vi "Merge Driver Call by Reference Error.vi"(8 "driver name":string, 10 "called vi error":errorcluster, 11 "call by ref error":errorcluster) -> (2 "error out":errorcluster)   [LabVIEW 2020, in "MeasurementLink Instrument.lvlib" / "ISession Factory.lvclass"]
uses:
  ISession Factory.lvclass
  MeasurementLink Measurement Server/Helpers/Error Strings Global Internal.vi
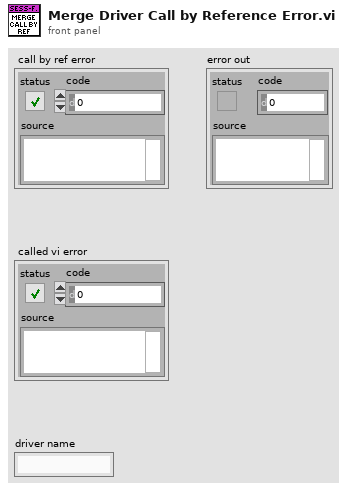
[diagram p1: front panel]
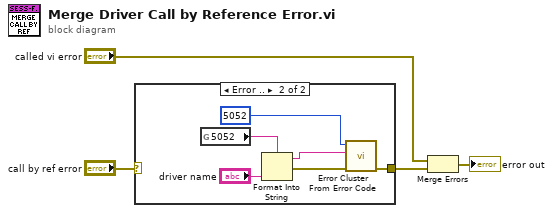
[diagram p0: block diagram]
diagram:
  n1 = case shown="Error .." "call by ref error" {
    selector: "call by ref error" -> [w5 _]
    tunnel: [w5 w6] -> w2
    frame No Error {
    }
    frame Error {
      n2 = global read "Error Strings Global Internal.vi" "5052"() -> (w9:string)
      n3 = Format Into String(format string=w9, "driver name") -> (resulting string=w10:string, error out=w11:errorcluster)  [unwired: 2 in]
      n4 = call <vilib>:"Error Cluster From Error Code.vi"("error in (no error)"=w11, "error message (\"\")"=w10, "error code (0)"=5052) -> ("error out"=w6:errorcluster)  [unwired: 6 in]
    }
  }
  n5 = Merge Errors("called vi error", w2) -> (→"error out":errorcluster)
